vi "split group into crates.vi"(0 "Group":T2 {"Channels in Group"."Card.Channel" format="%.2f"}, 7 "error in":errorcluster) -> (20 "Group Name":string, 21 "Channels in Crate 0":dbl[](array[numeric]), 22 "Num Channels in Crate 0":i32, 23 "Channels in Crate 1":dbl[](array[numeric]), 24 "Num Channels in Crate 1":i32, 25 "Channels in Crate 2":dbl[](array[numeric]), 26 "Num Channels in Crate 2":i32, 27 "error out":errorcluster)   [LabVIEW 2018]
uses:
  subvis/channel.ctl
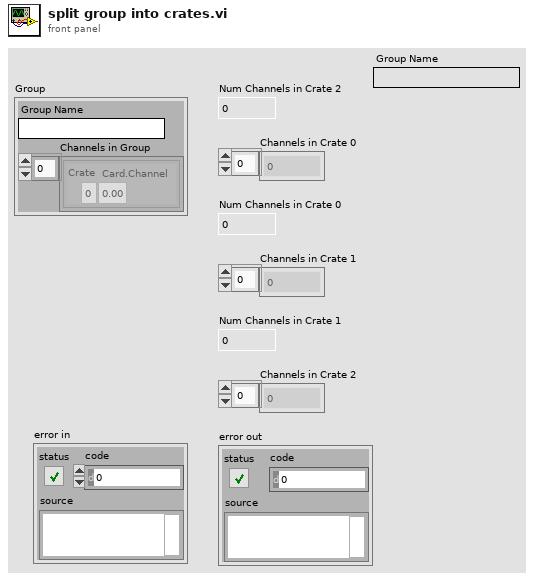
[diagram p1: front panel]
types:
  T1 = typedef "channel.ctl" = cluster{" Card.Channel":dbl, "Crate":i32}
  T2 = cluster{"Group Name":string, "Channels in Group":T1[]}
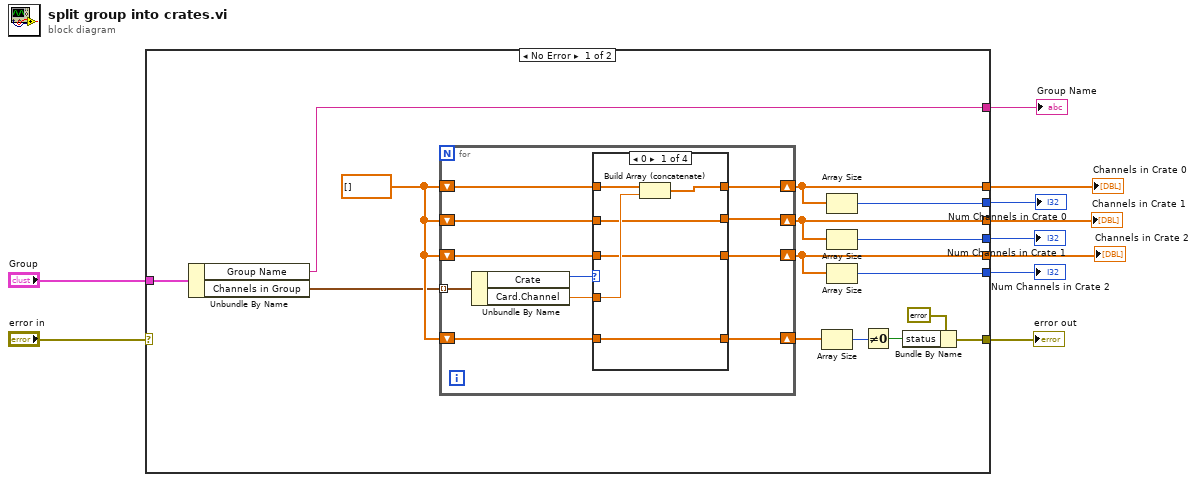
[diagram p0: block diagram]
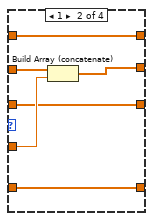
[diagram p2: hidden frame]
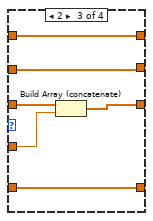
[diagram p3: hidden frame]
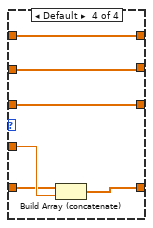
[diagram p4: hidden frame]
diagram:
  n1 = case shown="No Error" "error in" {
    selector: "error in" -> [_ w61]
    tunnel: [w25 _] -> w10
    tunnel: [w24 _] -> w9
    tunnel: [w23 _] -> w8
    tunnel: [w22 w61] -> w7
    tunnel: [w21 _] -> w6
    tunnel: [w20 _] -> w5
    tunnel: [w19 _] -> w4
    tunnel: "Group" -> [w12 _]
    tunnel: [w11 _] -> w2
    frame No Error {
      w14 = dbl[] []
      n2 = Unbundle By Name(w12) -> ("Group Name"=w11:string, "Channels in Group"=w13:T1[])
      n3 = for {
        tunnel: w13 -> [w36] mode=indexing
        shift-right: [w32] -> w19
        shift-left: w14 -> [w33]
        shift-right: [w31] -> w20
        shift-left: w14 -> [w30]
        shift-right: [w29] -> w21
        shift-left: w14 -> [w28]
        shift-right: [w27] -> w15
        shift-left: w14 -> [w26]
        n4 = Unbundle By Name(w36) -> ("Crate"=w35:i32, "Card.Channel"=w34:dbl)
        n5 = case shown="0" w35 {
          tunnel: w34 -> [w42 w48 w54 w60]
          tunnel: w33 -> [w41 w46 w50 w57]
          tunnel: [w40 w46 w50 w57] -> w32
          tunnel: [w39 w47 w51 w56] -> w31
          tunnel: w30 -> [w39 w45 w51 w56]
          tunnel: [w38 w44 w52 w55] -> w29
          tunnel: w28 -> [w38 w44 w53 w55]
          tunnel: [w37 w43 w49 w59] -> w27
          tunnel: w26 -> [w37 w43 w49 w58]
          frame 0 {
            n6 = Build Array (concatenate)(w41, w42) -> (w40:dbl[])
          }
          frame 1 {
            n7 = Build Array (concatenate)(w45, w48) -> (w47:dbl[])
          }
          frame 2 {
            n8 = Build Array (concatenate)(w53, w54) -> (w52:dbl[])
          }
          frame Default {
            n9 = Build Array (concatenate)(w58, w60) -> (w59:dbl[])
          }
        }
      }
      n10 = Array Size(array=w15) -> (size(s)=w16:i32)
      n11 = Array Size(array=w19) -> (size(s)=w23:i32)
      n12 = Array Size(array=w20) -> (size(s)=w25:i32)
      n13 = Array Size(array=w21) -> (size(s)=w24:i32)
      n14 = Not Equal To 0?(x=w16) -> (x != 0?=w18:bool)
      n15 = Bundle By Name(cluster=errorcluster {"status"=FALSE, "code"=0, "source"="Group contains channels in unrecognised crate number!"} ("error out"), "status"=w18) -> (w22:errorcluster)
    }
    frame Error {
    }
  }
  "Num Channels in Crate 1" <- w10
  "Num Channels in Crate 2" <- w9
  "Num Channels in Crate 0" <- w8
  "error out" <- w7
  "Channels in Crate 2" <- w6
  "Channels in Crate 1" <- w5
  "Channels in Crate 0" <- w4
  "Group Name" <- w2
